vi "NMR_Long_RF_Pulse_Sequence_V4.vi"() -> ()   [LabVIEW 2020]
uses:
  <instrlib>/niFgen/niFgen.llb/niFgen Output Mode.ctl
  <instrlib>/niFgen/niFgen.llb/niFgen Waveform Type.ctl
  <instrlib>/niFgen/niFgen.llb/niFgen_ctl Trigger DigEdge - Edge Values (Ring).ctl
  <instrlib>/niFgen/niFgen.llb/niFgen_ctl Trigger Source Values (Ring).ctl
  <instrlib>/niFgen/niFgen.llb/niFgen Trigger Mode.ctl
  <instrlib>/niScope/Controls/niScope acquisition type.ctl
  <instrlib>/niScope/Controls/niScope trigger slope.ctl
  <instrlib>/niScope/Controls/niScope trigger source.ctl
  <vilib>/Analysis/2dsp.llb/Integral Method.ctl
  <vilib>/Analysis/8numeric.llb/1D Numeric Integration.vi
  <vilib>/Utility/file.llb/Read Delimited Spreadsheet (DBL).vi
  <instrlib>/niFgen/niFgen.llb/niFgen Create Waveform (DBL).vi
  <instrlib>/niScope/Configure/Trigger/niScope Configure Trigger Edge.vi
  <instrlib>/niFgen/niFgen.llb/niFgen Configure Digital Edge Start Trigger.vi
  <instrlib>/niScope/Acquire/Fetch/niScope Fetch Cluster.vi
  <vilib>/Utility/file.llb/Write Delimited Spreadsheet (DBL).vi
  <vilib>/Analysis/NI_AALPro.lvlib
panel:
  out "Scan Number":i32
  out "Averaged T2 Decay":waveform(dbl)(graph) caption="Waveform Graph"
  out "Signal Intensity (Integral)":dbl format="%0.4f"
  out "output array":dbl[][](array[numeric])
  out "Extracted T2 Decay":waveform(dbl)(graph) caption="Waveform Graph"
  in  "Raw Waveform Data Output":path=path "C:/Users/localuser/OneDrive - University of South Carolina/NMR Research/Experimental Data & Pictures/Waveform.txt"
  out "Raw Waveform Data":T1(graph) caption="Waveform Graph"
  in  "resource name":refnum<k15>="PXI1Slot5" caption="ADC Conversion"
  in  "Sample Rate":dbl=12500000.0 caption="Pulse Sample Rate" format="%.2p"
  in  "FGEN Resource Name 2":refnum<k15>="FGEN2" caption="Pulse Generator"
  in  "Pulse Train File":path=path "C:/Users/localuser/OneDrive - University of South Carolina/NMR Research/Simulations/wfm.txt"
  in  "Larmor Frequency":dbl=27422000.0 caption="Frequency" format="%.4p"
  in  "Delay Time (ms)":u32=6000
  in  "Number of Scans":i32=1
  in  "Sine Wave Module":refnum<k15>="Dev1" caption="FGEN Resource Name"
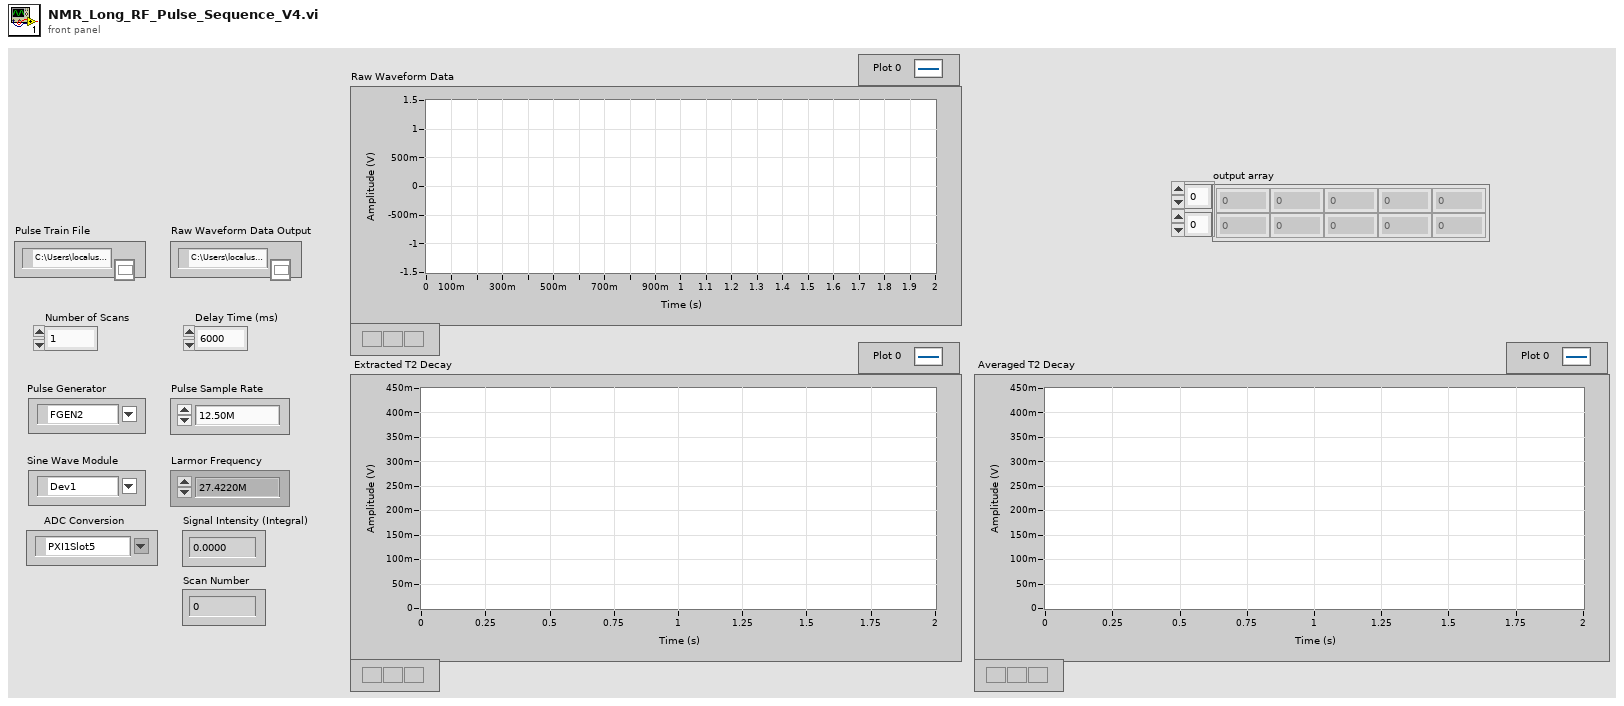
[diagram p1: front panel]
types:
  T1 = cluster{"relativeInitialX":dbl, "xIncrement":dbl, "wfm":dbl[]}
  T2 = typedef "niFgen Output Mode.ctl" = u32
  T3 = typedef "niScope trigger source.ctl" = string
  T4 = typedef "niFgen_ctl Trigger Source Values (Ring).ctl" = string
  T5 = typedef "NI_AALPro.lvlib/Integral Method.ctl" = i32
  T6 = typedef "niScope trigger slope.ctl" = i32
  T7 = typedef "niScope acquisition type.ctl" = i32
  T8 = typedef "niFgen Trigger Mode.ctl" = i32
  T9 = typedef "niFgen_ctl Trigger DigEdge - Edge Values (Ring).ctl" = i32
  T10 = typedef "niFgen Waveform Type.ctl" = i32
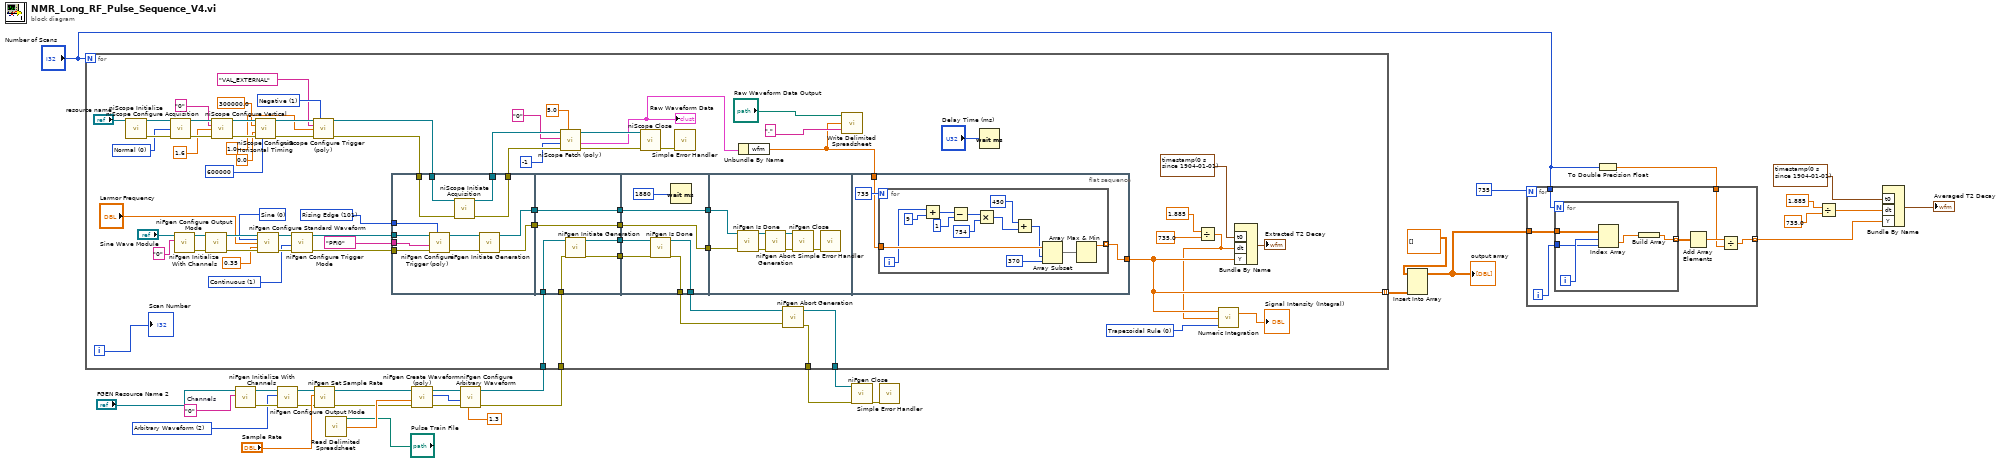
[diagram p0: block diagram]
diagram:
  w19 = "0"  # Channels
  w18 = T2 2 items=["Standard Function", "Frequency List", "Arbitrary Waveform", "Arbitrary Sequence", "Script"] ("output mode")
  n1 = call <instrlib>:"niFgen Initialize With Channels.vi"("Channel Name"=w19, "Resource Name"="FGEN Resource Name 2") -> ("error out"=w22:errorcluster, "Instrument Handle Out"=w23:refnum<k15>)  [unwired: 8 in]
  n2 = call <instrlib>:"niFgen Configure Output Mode.vi"("error in (no error)"=w22, "Output Mode (default: 0=Standard Function)"=w18, "Instrument Handle"=w23) -> ("error out"=w26:errorcluster, "Instrument Handle Out"=w25:refnum<k15>)  [unwired: 6 in]
  n3 = call <instrlib>:"niFgen Set Sample Rate.vi"("error in (no error)"=w26, "Sample Rate (Samp/s)"="Sample Rate", "Instrument Handle"=w25) -> ("error out"=w29:errorcluster, "Instrument Handle Out"=w28:refnum<k15>)  [unwired: 7 in]
  n4 = call-poly <vilib>:"Read Delimited Spreadsheet.vi"("file path (dialog if empty)"="Pulse Train File") -> ("first row"=w30:dbl[])  [unwired: 9 in, 5 out]
  n5 = call-poly <instrlib>:"niFgen Create Waveform (poly).vi"("error in (no error)"=w29, "Waveform Data Array"=w30, "Instrument Handle"=w28) -> ("error out"=w32:errorcluster, "Waveform Handle"=w33:i32, "Instrument Handle Out"=w31:refnum<k15>)  [unwired: 6 in]
  n6 = call <instrlib>:"niFgen Configure Arbitrary Waveform.vi"("Gain"=1.3, "error in (no error)"=w32, "Waveform Handle"=w33, "Instrument Handle"=w31) -> ("error out"=w17:errorcluster, "Instrument Handle Out"=w16:refnum<k15>)  [unwired: 6 in]
  n7 = for {
    N: "Number of Scans" -> [_]
    tunnel: w17 -> [w87]
    tunnel: w16 -> [w86]
    tunnel: [w85] -> w14
    tunnel: [w84] -> w13
    tunnel: [w38] -> w9 mode=indexing
    i -> [w34]
    w36 = T5 0 items=["Trapezoidal Rule", "Simpson's Rule", "Simpson's 3/8 Rule", "Bode Rule"] ("integration method")
    w72 = T6 1 items=["Positive", "Negative"] ("trigger slope")
    w73 = T7 0 items=["Normal"=0, "Flex Res"=1, "DDC"=3] ("acquisition Type")
    w92 = T8 1 items=["Single", "Continuous", "Stepped", "Burst"] ("Trigger Mode (default: 1=continuous)")
    w96 = T9 101 items=["Rising Edge"=101, "Falling Edge"=102] ("Edge (Rising)")
    w97 = T10 0 items=["Sine", "Square", "Triangle", "Ramp Up", "Ramp Down", "DC", "Noise", "User"] ("Waveform")
    n8 = call <instrlib>:"niScope Initialize.vi"("resource name"="resource name") -> ("instrument handle"=w74:refnum<k15>, "error out"=w75:errorcluster)  [unwired: 13 in]
    n9 = call <instrlib>:"niScope Configure Acquisition.vi"("instrument handle"=w74, "acquisition Type"=w73, "error in"=w75) -> ("instrument handle out"=w77:refnum<k15>, "error out"=w78:errorcluster)  [unwired: 11 in]
    n10 = call <instrlib>:"niFgen Initialize With Channels.vi"("Channel Name"="0", "Resource Name"="Sine Wave Module") -> ("error out"=w102:errorcluster, "Instrument Handle Out"=w105:refnum<k15>)  [unwired: 8 in]
    n11 = call <instrlib>:"niFgen Configure Output Mode.vi"("error in (no error)"=w102, "Instrument Handle"=w105) -> ("error out"=w101:errorcluster, "Instrument Handle Out"=w104:refnum<k15>)  [unwired: 7 in]
    n12 = call <instrlib>:"niScope Configure Vertical.vi"("instrument handle"=w77, "channels"="0", "vertical range"=1.6, "error in"=w78) -> ("instrument handle out"=w79:refnum<k15>, "error out"=w80:errorcluster)  [unwired: 10 in]
    n13 = call <instrlib>:"niScope Configure Horizontal Timing.vi"("instrument handle"=w79, "min sample rate"=300000.0, "reference position"=0.0, "error in"=w80, "min record length"=600000) -> ("instrument handle out"=w81:refnum<k15>, "error out"=w82:errorcluster)  [unwired: 9 in]
    n14 = call <instrlib>:"niFgen Configure Standard Waveform.vi"("Instrument Handle"=w104, "Waveform"=w97, "Frequency"="Larmor Frequency", "Amplitude"=0.35, "error in (no error)"=w101) -> ("Instrument Handle Out"=w103:refnum<k15>, "error out"=w100:errorcluster)  [unwired: 9 in]
    n15 = call <instrlib>:"niFgen Configure Trigger Mode.vi"("error in (no error)"=w100, "Trigger Mode (default: 1=continuous)"=w92, "Instrument Handle"=w103) -> ("error out"=w95:errorcluster, "Instrument Handle Out"=w93:refnum<k15>)  [unwired: 7 in]
    n16 = call-poly <instrlib>:"niScope Configure Trigger (poly).vi"("instrument handle"=w81, "trigger slope"=w72, "trigger source"=T3 "VAL_EXTERNAL", "trigger level"=1.0, "error in"=w82) -> ("instrument handle out"=w64:refnum<k15>, "error out"=w63:errorcluster)  [unwired: 9 in]
    n17 = flat-sequence {
      tunnel: w96 -> [w116]
      tunnel: w95 -> [w115]
      tunnel: T4 "PFI0" ("Source") -> [w114]
      tunnel: w93 -> [w113]
      tunnel: w64 -> [w111]
      tunnel: w63 -> [w110]
      tunnel: [w109] -> w62
      tunnel: [w108] -> w61
      tunnel: [w107] -> w46
      tunnel: [w106] -> w43
      tunnel: w87 -> [w123]
      tunnel: w86 -> [w122]
      tunnel: [w121] -> w50
      tunnel: [w120] -> w49
      tunnel: [w119] -> w47
      tunnel: w46 -> [w119]
      tunnel: [w118] -> w44
      tunnel: w43 -> [w118]
      tunnel: [w129] -> w90
      tunnel: [w128] -> w89
      tunnel: w50 -> [w127]
      tunnel: w49 -> [w126]
      tunnel: [w125] -> w48
      tunnel: w47 -> [w125]
      tunnel: [w124] -> w45
      tunnel: w44 -> [w124]
      tunnel: w48 -> [w132]
      tunnel: w45 -> [w131]
      tunnel: w52 -> [w139]
      tunnel: [w138] -> w38
      frame #0 {
        n18 = call-poly <instrlib>:"niFgen Configure Trigger (poly).vi"("Edge (Rising)"=w116, "error in (no error)"=w115, "Source"=w114, "Instrument Handle"=w113) -> ("error out"=w112:errorcluster, "Instrument Handle Out"=w117:refnum<k15>)  [unwired: 6 in]
        n19 = call <instrlib>:"niScope Initiate Acquisition.vi"("instrument handle"=w111, "error in"=w110) -> ("instrument handle out"=w109:refnum<k15>, "error out"=w108:errorcluster)  [unwired: 12 in]
        n20 = call <instrlib>:"niFgen Initiate Generation.vi"("error in (no error)"=w112, "Instrument Handle"=w117) -> ("error out"=w106:errorcluster, "Instrument Handle Out"=w107:refnum<k15>)  [unwired: 8 in]
      }
      frame #1 {
        n21 = call <instrlib>:"niFgen Initiate Generation.vi"("error in (no error)"=w123, "Instrument Handle"=w122) -> ("error out"=w120:errorcluster, "Instrument Handle Out"=w121:refnum<k15>)  [unwired: 8 in]
      }
      frame #2 {
        n22 = call <instrlib>:"niFgen Is Done.vi"("error in (no error)"=w126, "Instrument Handle"=w127) -> ("error out"=w129:errorcluster, "Instrument Handle Out"=w128:refnum<k15>)  [unwired: 7 in, 1 out]
        n23 = Wait (ms)(milliseconds to wait=u32 1880) -> ()  [unwired: 1 out]
      }
      frame #3 {
        n24 = call <instrlib>:"niFgen Is Done.vi"("error in (no error)"=w131, "Instrument Handle"=w132) -> ("error out"=w135:errorcluster, "Instrument Handle Out"=w134:refnum<k15>)  [unwired: 7 in, 1 out]
        n25 = call <instrlib>:"niFgen Abort Generation.vi"("error in (no error)"=w135, "Instrument Handle"=w134) -> ("error out"=w136:errorcluster, "Instrument Handle Out"=w137:refnum<k15>)  [unwired: 8 in]
        n26 = call <instrlib>:"niFgen Close.vi"("error in (no error)"=w136, "Instrument Handle"=w137) -> ("error out"=w133:errorcluster)  [unwired: 9 in]
        n27 = call <vilib>:"Simple Error Handler.vi"("error in (no error)"=w133) -> ()  [unwired: 4 in, 5 out]
      }
      frame #4 {
        n28 = for {
          N: 735 -> [_]
          tunnel: [w147] -> w138 mode=indexing
          tunnel: w139 -> [w146]
          i -> [w141]
          n29 = Add(x=w141, y=9) -> (x+y=w152:i32)
          n30 = Subtract(x=w152, y=1) -> (x-y=w150:i32)
          n31 = Multiply(x=w150, y=754) -> (x*y=w145:i32)
          n32 = Add(x=450, y=w145) -> (x+y=w143:i32)
          n33 = Array Subset(array=w146, index=w143, length=370 ("y")) -> (w148:dbl[])
          n34 = Array Max & Min(array=w148) -> (max value=w147:dbl)  [unwired: 3 out]
        }
      }
    }
    n35 = call-poly <instrlib>:"niScope Fetch (poly).vi"("timeout"=5.0, "error in"=w61, "numSamples"=-1, "channels"="0", "instrument handle"=w62) -> ("error out"=w58:errorcluster, "waveform"=w55:T1, "instrument handle out"=w57:refnum<k15>)  [unwired: 3 in, 1 out]
    "Raw Waveform Data" <- w55
    n36 = call <instrlib>:"niScope Close.vi"("instrument handle"=w57, "error in"=w58) -> ("error out"=w83:errorcluster)  [unwired: 13 in]
    n37 = call <vilib>:"Simple Error Handler.vi"("error in (no error)"=w83) -> ()  [unwired: 4 in, 5 out]
    n38 = Unbundle By Name(w55) -> ("wfm"=w52:dbl[])
    n39 = call <instrlib>:"niFgen Abort Generation.vi"("error in (no error)"=w90, "Instrument Handle"=w89) -> ("error out"=w85:errorcluster, "Instrument Handle Out"=w84:refnum<k15>)  [unwired: 8 in]
    n40 = call-poly <vilib>:"Write Delimited Spreadsheet.vi"("file path (dialog if empty)"="Raw Waveform Data Output", "1D data"=w52, "delimiter (\\t)"="," ("delimiter (\\t)")) -> ()  [unwired: 11 in, 2 out]
    n41 = Wait (ms)(milliseconds to wait="Delay Time (ms)") -> ()  [unwired: 1 out]
    n42 = Divide(x=1.885, y=735.0) -> (x/y=w37:dbl)
    n43 = call-poly <vilib>:"Numeric Integration.vi"("integration method"=w36, "dt"=w37, "Input Array"=w38) -> ("result"=→"Signal Intensity (Integral)":dbl)  [unwired: 1 out]
    n44 = Bundle By Name("t0"=timestamp(0 s since 1904-01-01), "dt"=w37, "Y"=w38) -> (→"Extracted T2 Decay":waveform(dbl))  [unwired: 1 in]
    "Scan Number" <- w34
  }
  n45 = call <instrlib>:"niFgen Close.vi"("error in (no error)"=w14, "Instrument Handle"=w13) -> ("error out"=w15:errorcluster)  [unwired: 9 in]
  n46 = call <vilib>:"Simple Error Handler.vi"("error in (no error)"=w15) -> ()  [unwired: 4 in, 5 out]
  n47 = Insert Into Array(array=dbl[][] [], new element=w9) -> (w12:dbl[][])  [unwired: 2 in]
  "output array" <- w12
  n48 = To Double Precision Float(number="Number of Scans") -> (double precision float=w8:dbl)
  n49 = for {
    N: 735 -> [_]
    tunnel: w12 -> [w160]
    tunnel: [w156] -> w2 mode=indexing
    tunnel: "Number of Scans" -> [w155]
    tunnel: w8 -> [w154]
    i -> [w159]
    n50 = for {
      N: w155 -> [_]
      tunnel: w160 -> [w165]
      tunnel: w159 -> [w163]
      tunnel: [w161] -> w158 mode=indexing
      i -> [w164]
      n51 = Index Array(array=w165, index (row)=w164, index (col)=w163) -> (element=w162:dbl)
      n52 = Build Array(w162) -> (w161:dbl[])
    }
    n53 = Add Array Elements(numeric array=w158) -> (sum=w157:dbl)
    n54 = Divide(x=w157, y=w154) -> (x/y=w156:dbl)
  }
  n55 = Divide(x=1.885, y=735.0) -> (x/y=w3:dbl)
  n56 = Bundle By Name("t0"=timestamp(0 s since 1904-01-01), "dt"=w3, "Y"=w2) -> (→"Averaged T2 Decay":waveform(dbl))  [unwired: 1 in]
